vi "Write UI Object.vi"(8 "error in (no error)":errorcluster, 10 "Flex UI in":refnum<class "Flex UI.lvclass">, 11 "Flex UI (Actor) in":refnum<class "Flex UI (Actor).lvclass">) -> (0 "error out":errorcluster, 3 "Flex UI (Actor) out":refnum<class "Flex UI (Actor).lvclass">)   [LabVIEW 2016, in "Flex UI (Parent Actor).lvlib" / "Flex UI (Actor).lvclass"]
uses:
  Flex UI (Actor).lvclass
  <vilib>/East West Architects/Flex UI/Flex UI (Parent)/Flex UI.lvclass
  Flex UI (Actor).lvclass/Flex UI (Actor).ctl
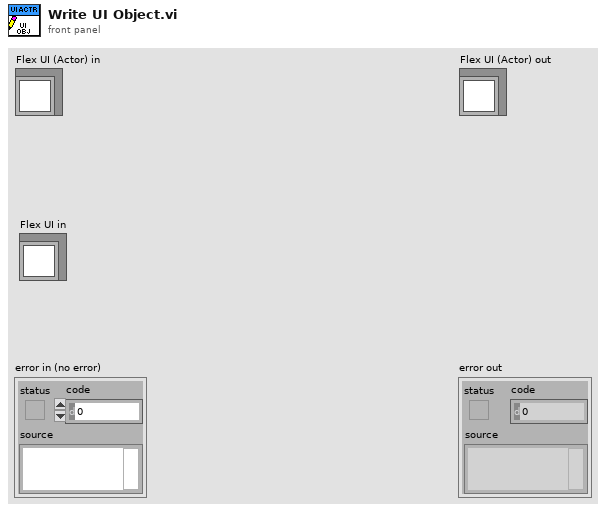
[diagram p1: front panel]
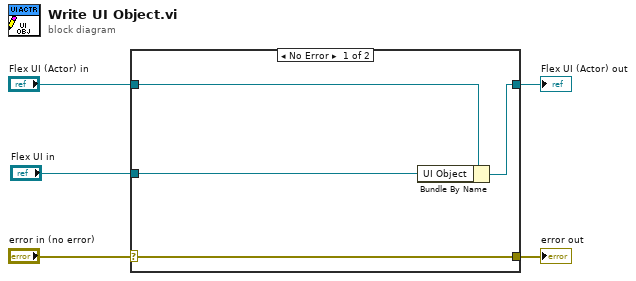
[diagram p0: block diagram]
diagram:
  n1 = case shown="No Error" "error in (no error)" {
    selector: "error in (no error)" -> [w9 w10]
    tunnel: [w9 w10] -> w4
    tunnel: [w7 w11] -> w2
    tunnel: "Flex UI (Actor) in" -> [w8 w11]
    tunnel: "Flex UI in" -> [w6 _]
    frame No Error {
      n2 = Bundle By Name(cluster=w8, "UI Object"=w6) -> (w7:refnum<class "Flex UI (Actor).lvclass">)
    }
    frame Error {
    }
  }
  "error out" <- w4
  "Flex UI (Actor) out" <- w2
